vi "Command Loop - Get HW Values.vi"(8 "error in":errorcluster, 10 "Data":string, 11 "Queue Refs in":T1) -> (0 "error out":errorcluster, 2 "Response":string, 3 "Queue Refs out":T1)   [LabVIEW 2025, in "Runtime Configuration Support Example Engine.lvlib"]
uses:
  Runtime Configuration Support Example Engine.lvlib
  Shared/Compiled.Settings.ctl
  <vilib>/NI VeriStand/Custom Device API/Custom Device Item Ref.ctl
  <vilib>/NI VeriStand/Custom Device API/Custom Device API.lvlib
  Shared/Runtime Configuration Support Example Shared.lvlib
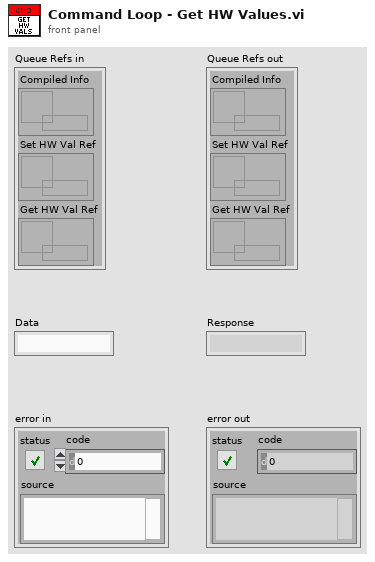
[diagram p1: front panel]
types:
  T1 = cluster{"Compiled Info":refnum<queue>, "Set HW Val Ref":refnum<queue>, "Get HW Val Ref":refnum<queue>}
  T2 = cluster{"In Indices":i32[], "Out Indices":i32[], "In Values":i32[], "Out Values":i32[], "Error":errorcluster}
  T3 = cluster{"SignalIDs In":i32[], "SignalIDs Out":i32[], "Response Ref":refnum<queue>}
  T4 = cluster{"SignalIDsIn":i32[], "SignalIDsOut":i32[]}
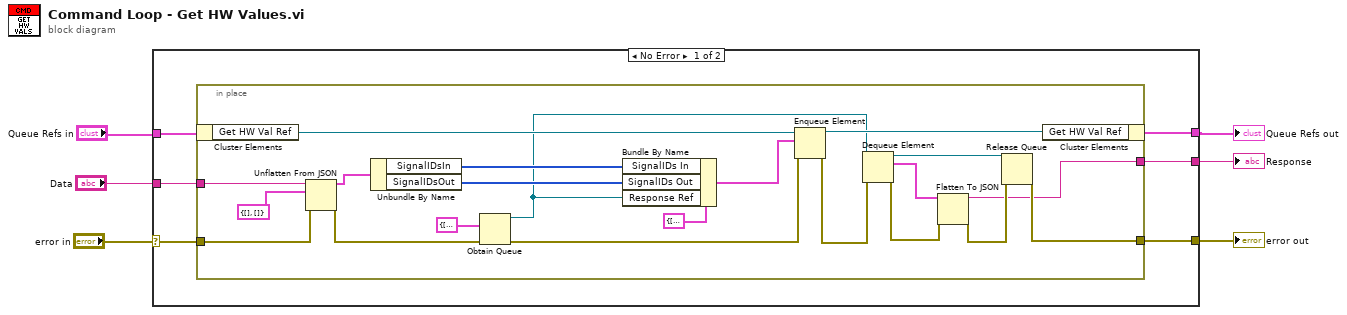
[diagram p0: block diagram]
diagram:
  n1 = case shown="No Error" "error in" {
    selector: "error in" -> [w12 w35]
    tunnel: "Data" -> [w10 _]
    tunnel: "Queue Refs in" -> [w9 w34]
    tunnel: [w11 w35] -> w5
    tunnel: [w8 _] -> w3
    tunnel: [w7 w34] -> w1
    frame No Error {
      n2 = in-place {
        in-place-border: w12 -> [w33]
        in-place-border: [w31] -> w11
        in-place-border: w10 -> [w14]
        in-place-border: [w23] -> w8
        n3 = in-place-cluster #1(w9) -> ("Get HW Val Ref"=w25:refnum<queue>)
        n4 = Unflatten From JSON(JSON string=w14, type and defaults=T4 {"SignalIDsIn"=[], "SignalIDsOut"=[]} ("Cluster"), error in (no error)=w33) -> (value=w19:T4, error out=w28:errorcluster)  [unwired: 4 in]
        n5 = Unbundle By Name(w19) -> ("SignalIDsIn"=w18:i32[], "SignalIDsOut"=w17:i32[])
        n6 = Obtain Queue(element data type=T2 {"In Indices"=[], "Out Indices"=[], "In Values"=[], "Out Values"=[], "Error"={"status"=FALSE, "code"=0, "source"=""}}, error in (no error)=w28) -> (queue out=w13:refnum<queue>, error out=w29:errorcluster)  [unwired: 3 in, 1 out]
        n7 = Bundle By Name(cluster=T3 {"SignalIDs In"=[], "SignalIDs Out"=[], "Response Ref"=refnum}, "SignalIDs In"=w18, "SignalIDs Out"=w17, "Response Ref"=w13) -> (w15:T3)
        n8 = Enqueue Element(queue=w25, element=w15, error in (no error)=w29) -> (queue out=w24:refnum<queue>, error out=w27:errorcluster)  [unwired: 1 in, 1 out]
        n9 = Dequeue Element(queue=w13, error in (no error)=w27) -> (queue out=w22:refnum<queue>, element=w26:T2, error out=w30:errorcluster)  [unwired: 1 in, 1 out]
        n10 = Flatten To JSON(anything=w26, error in (no error)=w30) -> (JSON string=w23:string, 11:w32:errorcluster)  [unwired: 1 in]
        n11 = Release Queue(queue=w22, error in (no error)=w32) -> (error out=w31:errorcluster)  [unwired: 1 in, 2 out]
        n12 = in-place-cluster #1("Get HW Val Ref"=w24) -> (w7:T1)
      }
    }
    frame Error {
    }
  }
  "error out" <- w5
  "Response" <- w3
  "Queue Refs out" <- w1
